vi "M2p_AD_Fifo.vi"() -> ()   [LabVIEW 2015]
uses:
  spcm_library/spcm_gui_common.llb/element_device.ctl
  spcm_library/spcm_gui_common.llb/element_mode_fifo.ctl
  spcm_library/spcm_gui_common.llb/element_device_infos.ctl
  spcm_library/spcm_gui_m2p.llb/element_m2p_ai_channel.ctl
  spcm_library/spcm_gui_m2p.llb/element_m2p_clock.ctl
  spcm_library/spcm_gui_m2p.llb/element_m2p_ai_trigger.ctl
panel:
  out "Display Ch2-Ch3":sgl[][](graph)
  out "Display Ch0-Ch1":sgl[][](graph)
  in  "Trigger Settings":T1={"Trigger Source"=0, "External Trigger"=0, "Level 0 Ext"=1500, "Ext Trig Term"=FALSE, "Channel Trigger"=0, "Level 0 Ch"=0, "Level 1 Ch"=0, "Trigger Delay (Samples)"=0} {"Channel Trigger" items=["None", "Pos. Edge", "Neg. Edge", "Any Edge", "Pos. Rearm", "Neg. Rearm", "Enter Window", "Leave Window", "In Win", "Out Win"]; "External Trigger" items=["None", "Pos. Edge", "Neg. Edge", "Any Edge", "High Level", "Low Level"]; "Trigger Source" items=["Software Trigger", "External Trigger", "Channel 0 Trigger", "Channel 1 Trigger", "Channel 2 Trigger", "Channel 3 Trigger", "Channel 4 Trigger", "Channel 5 Trigger", "Channel 6 Trigger", "Channel 7 Trigger"]; "Trigger Delay (Samples)" max=65535 step=1}
  in  "Clock Settings":T2={"Clock Mode"=0, "Sampling Rate (kHz)"=10000.0, "Clock Output"=FALSE, "Termination"=FALSE, "Ref. Clock (MHz)"=10.0, "Threshold (mV)"=1500} {"Threshold (mV)" min=-5000 max=5000; "Clock Mode" items=["Internal Clock Quartz", "External Clock", "External Reference Clock"]; "Ref. Clock (MHz)" min=0.0 max=125000.0; "Sampling Rate (kHz)" min=1.0 max=5000000.0}
  in  "AI Channel 7":T3={"Enable"=TRUE, "Input Range "=2, "Termination"=0, "Input Type"=0, "Offset"=0} {"Input Type" items=["Single-ended", "Differential"]; "Termination" items=["1 MOhm", "50 Ohm"]; "Input Range" items=["±200 mV", "±500 mV", "±1000 mV", "±2000 mV", "±5000 mV", "±10000 mV"]}
  in  "AI Channel 6":T3={"Enable"=TRUE, "Input Range "=2, "Termination"=0, "Input Type"=0, "Offset"=0} {"Input Type" items=["Single-ended", "Differential"]; "Termination" items=["1 MOhm", "50 Ohm"]; "Input Range" items=["±200 mV", "±500 mV", "±1000 mV", "±2000 mV", "±5000 mV", "±10000 mV"]}
  in  "AI Channel 5":T3={"Enable"=TRUE, "Input Range "=2, "Termination"=0, "Input Type"=0, "Offset"=0} {"Input Type" items=["Single-ended", "Differential"]; "Termination" items=["1 MOhm", "50 Ohm"]; "Input Range" items=["±200 mV", "±500 mV", "±1000 mV", "±2000 mV", "±5000 mV", "±10000 mV"]}
  in  "AI Channel 4":T3={"Enable"=TRUE, "Input Range "=2, "Termination"=0, "Input Type"=0, "Offset"=0} {"Input Type" items=["Single-ended", "Differential"]; "Termination" items=["1 MOhm", "50 Ohm"]; "Input Range" items=["±200 mV", "±500 mV", "±1000 mV", "±2000 mV", "±5000 mV", "±10000 mV"]}
  in  "AI Channel 3":T3={"Enable"=TRUE, "Input Range "=2, "Termination"=0, "Input Type"=0, "Offset"=0} {"Input Type" items=["Single-ended", "Differential"]; "Termination" items=["1 MOhm", "50 Ohm"]; "Input Range" items=["±200 mV", "±500 mV", "±1000 mV", "±2000 mV", "±5000 mV", "±10000 mV"]}
  in  "AI Channel 2":T3={"Enable"=TRUE, "Input Range "=2, "Termination"=0, "Input Type"=0, "Offset"=0} {"Input Type" items=["Single-ended", "Differential"]; "Termination" items=["1 MOhm", "50 Ohm"]; "Input Range" items=["±200 mV", "±500 mV", "±1000 mV", "±2000 mV", "±5000 mV", "±10000 mV"]}
  in  "AI Channel 1":T3={"Enable"=TRUE, "Input Range "=2, "Termination"=0, "Input Type"=0, "Offset"=0} {"Input Type" items=["Single-ended", "Differential"]; "Termination" items=["1 MOhm", "50 Ohm"]; "Input Range" items=["±200 mV", "±500 mV", "±1000 mV", "±2000 mV", "±5000 mV", "±10000 mV"]}
  in  "AI Channel 0":T3={"Enable"=TRUE, "Input Range "=2, "Termination"=0, "Input Type"=0, "Offset"=0} {"Input Type" items=["Single-ended", "Differential"]; "Termination" items=["1 MOhm", "50 Ohm"]; "Input Range" items=["±200 mV", "±500 mV", "±1000 mV", "±2000 mV", "±5000 mV", "±10000 mV"]}
  out "Device Infos":T4={"Device Name"="M2p.5942-x4", "Serial Number"=666.0, "Mem (MB)"=1024.0}
  out "Display Ch6-Ch7":sgl[][](graph)
  out "Display Ch4-Ch5":sgl[][](graph)
  in  "Mode Setup":T5={"Mode"=0, "Loop"=0, "Seg"=1024, "Post"=8192, "Pre"=32, "ABA"=16} {"Mode" items=["Singleshot", "Multiple Recording", "Gated Sampling", "ABA Mode"]; "ABA" min=2 max=65535 step=1; "Post" min=4 step=4; "Loop" min=8 step=4; "Pre" min=4 max=8176 step=4; "Seg" min=8 step=4}
  in  "Device":T6 {"Device" items=["Card", "digitizerNETBOX"]}
  out "Fillsize Fifo":i32(slide)=62 scale=0.0..1000.0
  out "Status":string="Stopped"
  in  "Quit Button":bool
  in  "Force Trigger Button":bool
  in  "Start Button":bool
  in  "Stop Button":bool
  # "M2p AD FIFO Example"
  # "Mode Settings"
  # "Range"
  # "Term"
  # "Type"
  # "Offset"
  # "Ch0"
  # "Ch1"
  # "Clock Settings"
  # "Ch2"
  # "Ch3"
  # "Ch4"
  # "Trigger Settings"
  # "Ch5"
  # "Ch6"
  # "Ch7"
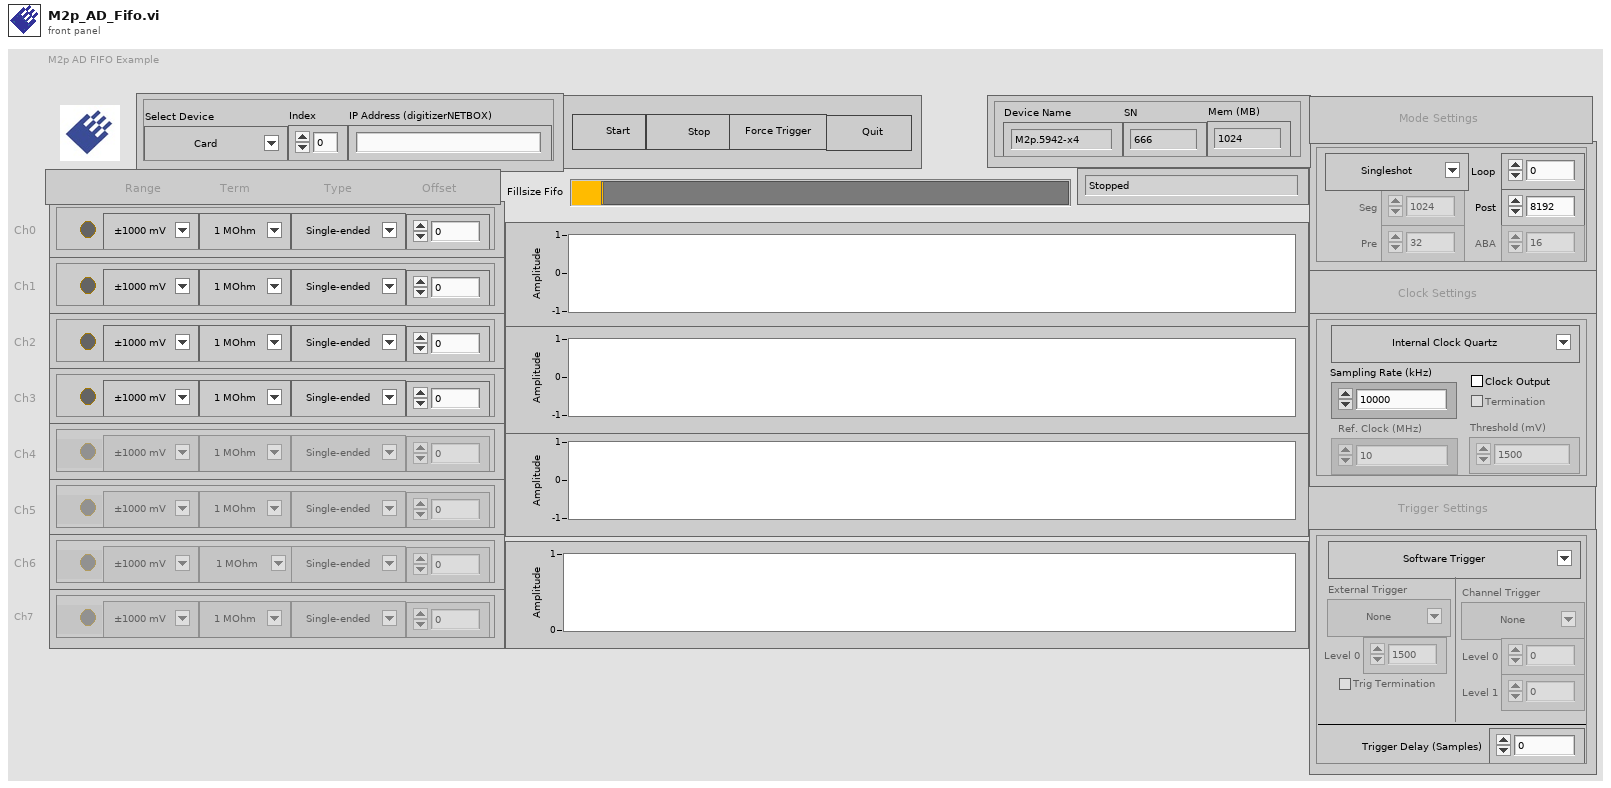
[diagram p1: front panel]
types:
  T1 = typedef "element_m2p_ai_trigger.ctl" = cluster{"Trigger Source":u16, "External Trigger":u16, "Level 0 Ext":i32, "Ext Trig Term":bool, "Channel Trigger":u16, "Level 0 Ch":i32, "Level 1 Ch":i32, "Trigger Delay (Samples)":u32}
  T2 = typedef "element_m2p_clock.ctl" = cluster{"Clock Mode":u16, "Sampling Rate (kHz)":dbl, "Clock Output":bool, "Termination":bool, "Ref. Clock (MHz)":dbl, "Threshold (mV)":i32}
  T3 = typedef "element_m2p_ai_channel.ctl" = cluster{"Enable":bool, "Input Range ":u16, "Termination":u16, "Input Type":u16, "Offset":i32}
  T4 = typedef "element_device_infos.ctl" = cluster{"Device Name":string, "Serial Number":dbl, "Mem (MB)":dbl}
  T5 = typedef "element_mode_fifo.ctl" = cluster{"Mode":u16, "Loop":u32, "Seg":u32, "Post":u32, "Pre":u32, "ABA":u32}
  T6 = typedef "element_device.ctl" = cluster{"Index":dbl, "IP Address":string, "Device":u16}
  T7 = enum16{"Idle", "Init", "Stop", "Write Setup", "Start", "Acquire", "Read Data", "Quit"}
  T8 = cluster{"Card Type":i32, "Inst Mem (high part)":i32, "Inst Mem (low part)":i32, "Serial Number":i32, "Function Type":i32, "Installed Features":i32, "Base Card Version":i32, "Module Version":i32, "Extension Version":i32, "Production Date":i32, "Max Sampling Rate":i32, "Max Channels":i32, "Demo Card":i32}
  T9 = cluster{"Card Name":string, "SN":i32, "Mem (MB)":i32}
  T10 = cluster{"AI Channels":i32, "AI Ranges":i32, "Input Ranges (mV)":i32[], "Programmable Offset":i32, "Termination Available":bool, "SE/Diff switchable":bool, "Offset in per cent/mV":bool, "Offset Calibration":bool, "Gain Calibration":bool, "Offset with open inputs":bool, "AI Range Strings[]":string[], "Bit Resolution":i32, "AC Coupling available":bool, "BW Limit available":bool, "AI Path count":i32}
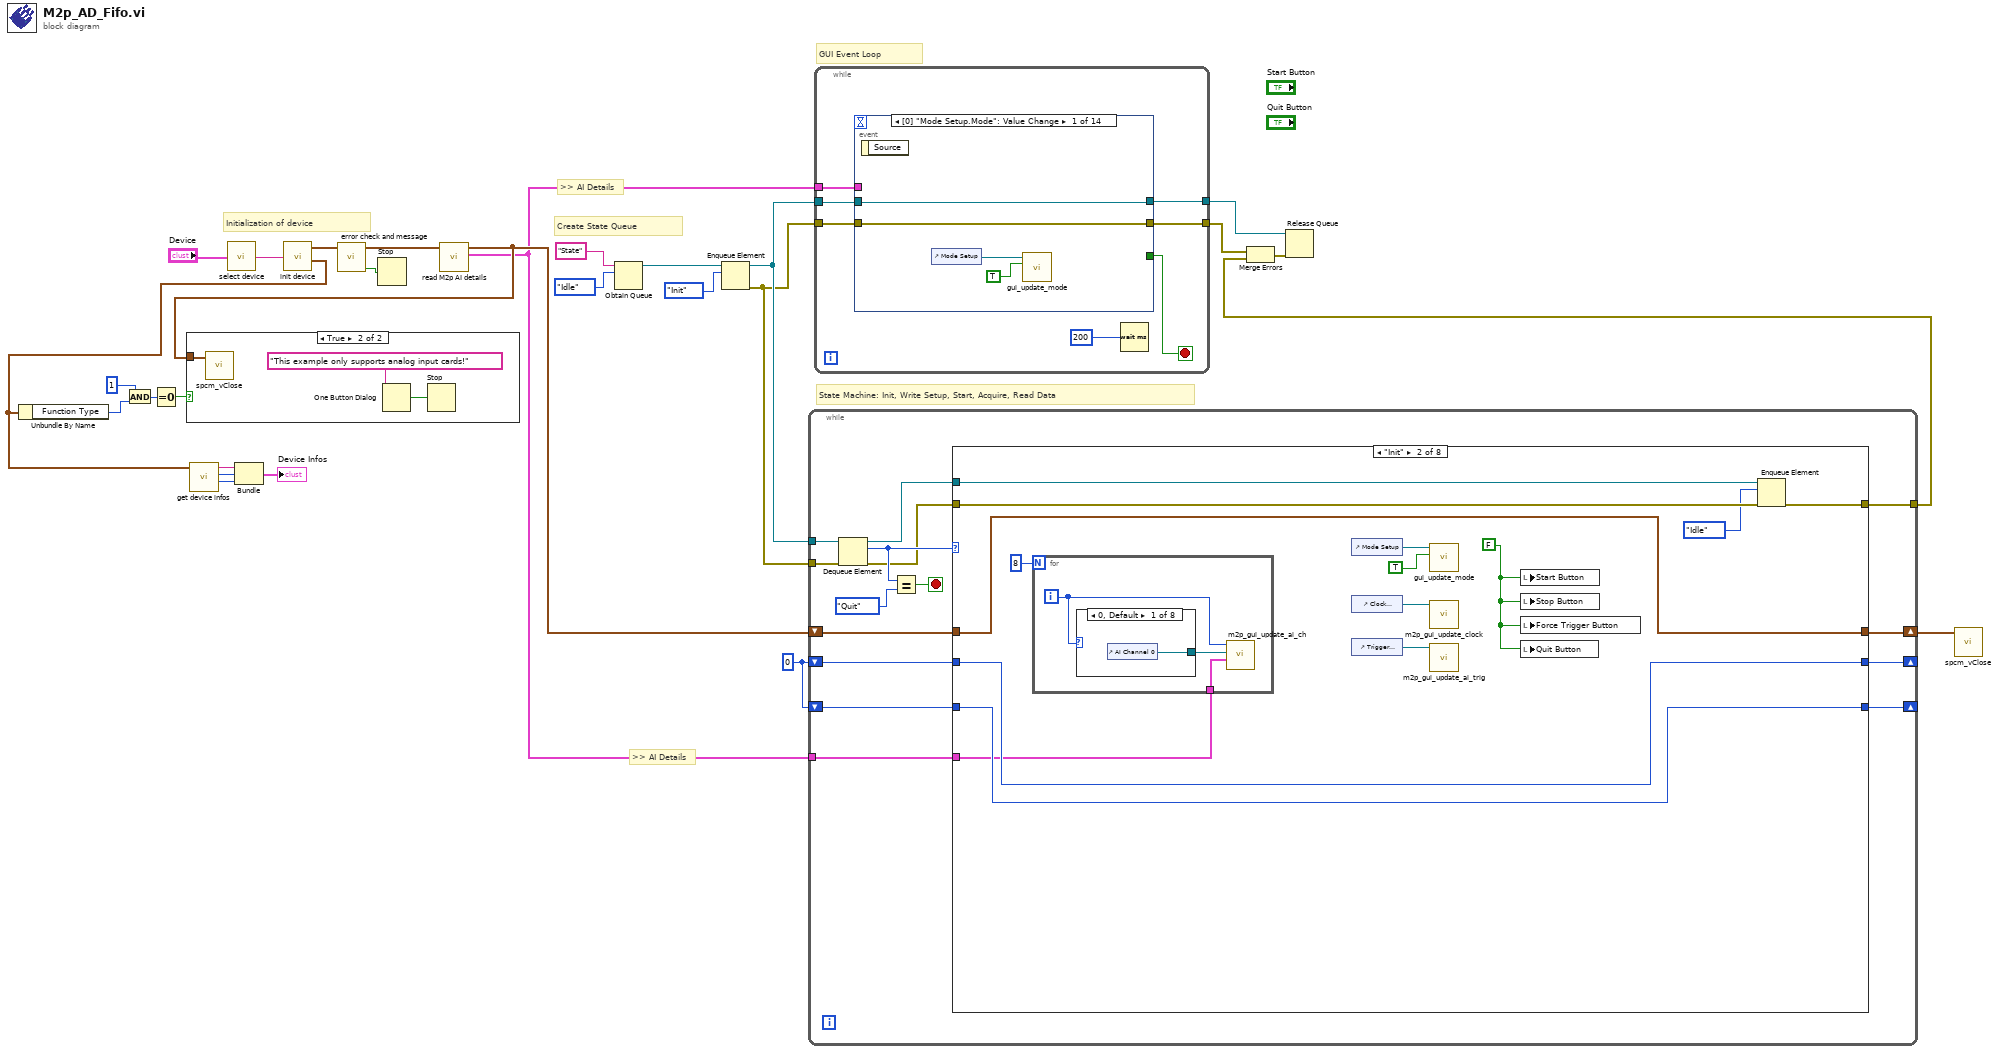
[diagram p0: block diagram]
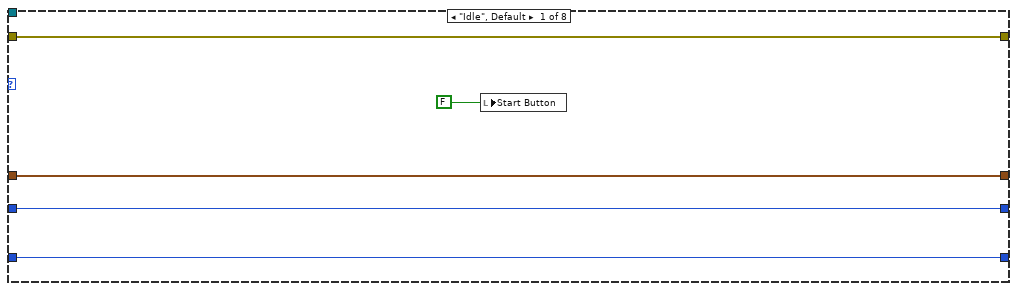
[diagram p3: hidden frame]
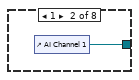
[diagram p4: hidden frame]
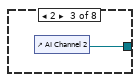
[diagram p5: hidden frame]
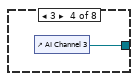
[diagram p6: hidden frame]
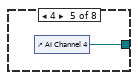
[diagram p7: hidden frame]
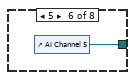
[diagram p8: hidden frame]
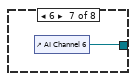
[diagram p9: hidden frame]
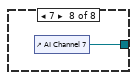
[diagram p10: hidden frame]
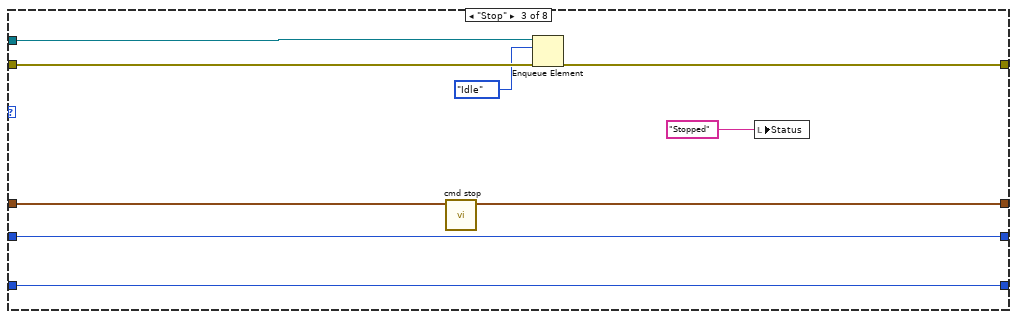
[diagram p11: hidden frame]
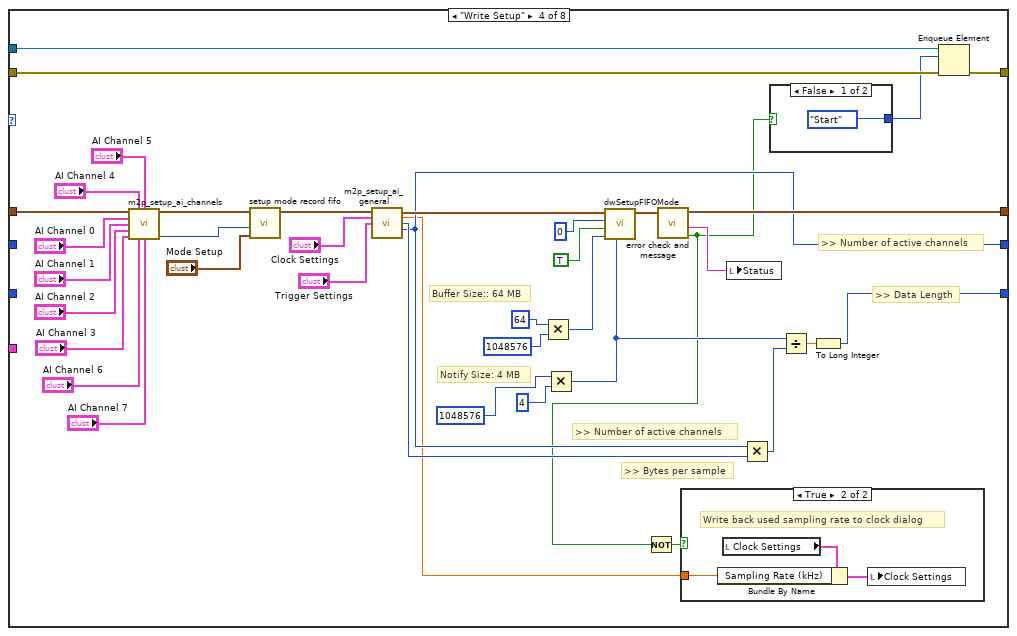
[diagram p12: hidden frame]
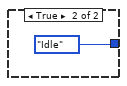
[diagram p14: hidden frame]
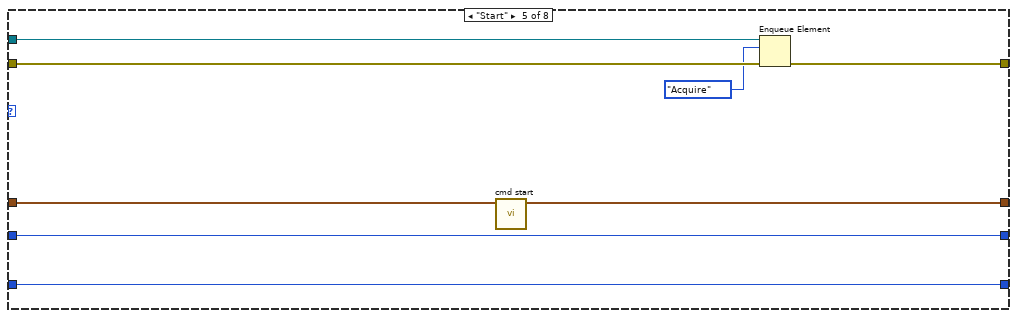
[diagram p15: hidden frame]
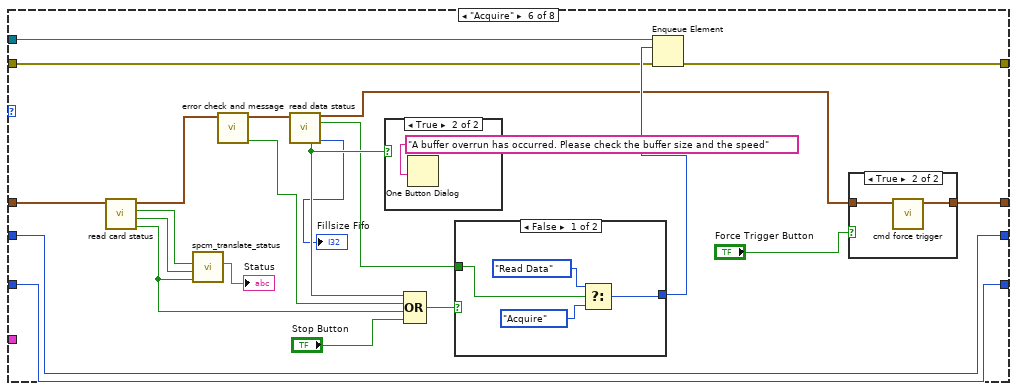
[diagram p16: hidden frame]
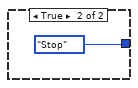
[diagram p18: hidden frame]
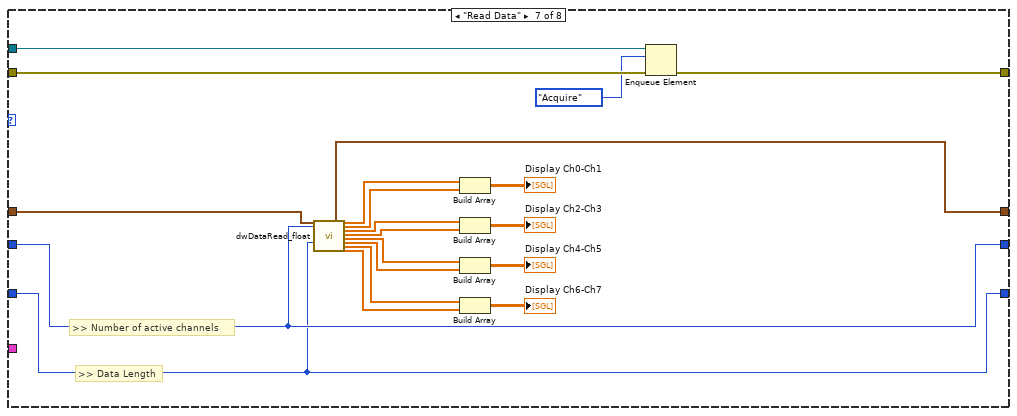
[diagram p20: hidden frame]
diagram:
  w6 = 0
  # ">> AI Details"
  # ">> AI Details"
  # "Initialization of device"
  # "Create State Queue"
  # "State Machine: Init, Write Setup, Start, Acquire, Read Data"
  # "GUI Event Loop"
  n1 = call "select device.vi"("Device"="Device") -> ("device string"=w28:string)  [unwired: 4 in]
  n2 = call "init device.vi"("Device String"=w28) -> ("Card Info Out"=w27:cluster{"Card Handle":u64, "Error Code":u32}, "Card Information"=w14:T8)  [unwired: 4 in]
  n3 = Unbundle By Name(w14) -> ("Function Type"=w18:i32)
  n4 = And(x=1, y=w18) -> (x .and. y?=w17:i32)
  n5 = Equal To 0?(x=w17) -> (x = 0?=w15:bool)
  n6 = call "get device infos.vi"("Card Information"=w14) -> ("Mem (MB)"=w21:i32, "SN"=w20:i32, "Card Name"=w19:string)  [unwired: 8 in]
  n7 = Bundle("Card Name"=w19, "SN"=w20, "Mem (MB)"=w21) -> (→"Device Infos":T9)  [unwired: 1 in]
  n8 = call "error check and message.vi"("Card Info In"=w27) -> ("Error occurred"=w26:bool, "Card Info Out"=w4:cluster{"Card Handle":u64, "Error Code":u32})  [unwired: 4 in, 1 out]
  n9 = Stop(stop? (T)=w26) -> ()
  n10 = call "read M2p AI details.vi"("Card Info In"=w4) -> ("AI Details"=w2:T10, "Card Info Out"=w3:cluster{"Card Handle":u64, "Error Code":u32})  [unwired: 5 in]
  n11 = case shown="True" w15 {
    tunnel: w3 -> [_ w29]
    frame False {
    }
    frame True {
      n12 = call "spcm_vClose.vi"("Card Info In"=w29) -> ()  [unwired: 7 in]
      n13 = One Button Dialog(message="This example only supports analog input cards!") -> (true=w30:bool)  [unwired: 1 in]
      n14 = Stop(stop? (T)=w30) -> ()
    }
  }
  n15 = Obtain Queue(name (unnamed)="State", element data type=T7."Idle") -> (queue out=w23:refnum<queue>)  [unwired: 3 in, 2 out]
  n16 = Enqueue Element(queue=w23, element=T7."Init") -> (queue out=w24:refnum<queue>, error out=w9:errorcluster)  [unwired: 2 in, 1 out]
  n17 = while {
    tunnel: w24 -> [w46]
    shift-right: [w44] -> w22
    shift-left: w3 -> [w45]
    shift-right: [w39] -> _
    shift-left: w6 -> [w40]
    tunnel: [w38] -> w12
    tunnel: w9 -> [w37]
    shift-right: [w34] -> _
    shift-left: w6 -> [w33]
    tunnel: w2 -> [w32]
    stop <- w42 stop-if-true
    n18 = Dequeue Element(queue=w46, error in (no error)=w37) -> (queue out=w41:refnum<queue>, element=w43:T7, error out=w36:errorcluster)  [unwired: 1 in, 1 out]
    n19 = Equal?(x=w43, y=T7."Quit") -> (x = y?=w42:bool)
    n20 = case shown="\"Init\"" w43 {
      tunnel: w45 -> [w51 w58 w82 w99 w136 w149 w187 w190]
      tunnel: [w51 w58 w81 w121 w135 w156 w181 w189] -> w44
      tunnel: w41 -> [_ w65 w85 w124 w133 w154 w188 _]
      tunnel: w40 -> [w50 w59 w80 _ w137 w153 w186 w194]
      tunnel: [w50 w59 w80 w102 w137 w153 w186 w194] -> w39
      tunnel: [w49 w63 w83 w122 w132 w151 w185 w195] -> w38
      tunnel: w36 -> [w49 w62 w84 w123 w134 w150 w184 w195]
      tunnel: [w47 w60 w79 w111 w130 w139 w183 w193] -> w34
      tunnel: w33 -> [w47 w60 w79 _ w130 w139 w183 w193]
      tunnel: w32 -> [_ w55 _ _ _ _ _ _]
      frame "Idle", Default {
        n21 = local write "Start Button"(FALSE) -> ()
      }
      frame "Init" {
        w64 = FALSE
        n22 = for {
          N: 8 -> [_]
          tunnel: w55 -> [w66]
          i -> [w68]
          n23 = case shown="0, Default" w68 {
            tunnel: [w69 w70 w71 w72 w73 w74 w75 w76] -> w67
            frame 0, Default {
              n24 = control-ref of="AI Channel 0"() -> (w69:refnum<vi>)
            }
            frame 1 {
              n25 = control-ref of="AI Channel 1"() -> (w70:refnum<vi>)
            }
            frame 2 {
              n26 = control-ref of="AI Channel 2"() -> (w71:refnum<vi>)
            }
            frame 3 {
              n27 = control-ref of="AI Channel 3"() -> (w72:refnum<vi>)
            }
            frame 4 {
              n28 = control-ref of="AI Channel 4"() -> (w73:refnum<vi>)
            }
            frame 5 {
              n29 = control-ref of="AI Channel 5"() -> (w74:refnum<vi>)
            }
            frame 6 {
              n30 = control-ref of="AI Channel 6"() -> (w75:refnum<vi>)
            }
            frame 7 {
              n31 = control-ref of="AI Channel 7"() -> (w76:refnum<vi>)
            }
          }
          n32 = call "m2p_gui_update_ai_ch.vi"("AI Details"=w66, "Cluster Referenz"=w67, "Channel Index"=w68) -> ()  [unwired: 9 in]
        }
        n33 = control-ref of="Mode Setup"() -> (w57:refnum<vi>)
        n34 = control-ref of="Clock Settings"() -> (w54:refnum<vi>)
        n35 = control-ref of="Trigger Settings"() -> (w53:refnum<vi>)
        n36 = call "gui_update_mode.vi"("Fifo Mode"=TRUE, "Referenz Mode Settings"=w57) -> ()  [unwired: 10 in]
        n37 = call "m2p_gui_update_clock.vi"("Cluster Reference"=w54) -> ()  [unwired: 11 in]
        n38 = call "m2p_gui_update_ai_trig.vi"("Trigger Settings Reference"=w53) -> ()  [unwired: 10 in]
        n39 = local write "Start Button"(w64) -> ()
        n40 = local write "Stop Button"(w64) -> ()
        n41 = local write "Force Trigger Button"(w64) -> ()
        n42 = local write "Quit Button"(w64) -> ()
        n43 = Enqueue Element(queue=w65, element=T7."Idle", error in (no error)=w62) -> (error out=w63:errorcluster)  [unwired: 1 in, 2 out]
      }
      frame "Stop" {
        n44 = call "cmd stop.vi"("Card Info In"=w82) -> ("Card Info Out"=w81:cluster{"Card Handle":u64, "Error Code":u32})  [unwired: 6 in]
        n45 = Enqueue Element(queue=w85, element=T7."Idle", error in (no error)=w84) -> (error out=w83:errorcluster)  [unwired: 1 in, 2 out]
        n46 = local write "Status"("Stopped") -> ()
      }
      frame "Write Setup" {
        # ">> Data Length"
        # ">> Number of active channels"
        # ">> Bytes per sample"
        # ">> Number of active channels"
        # "Buffer Size:: 64 MB"
        # "Notify Size: 4 MB"
        n47 = call "m2p_setup_ai_channels.vi"("Card Info In"=w99, "AI Channel 4"="AI Channel 4", "AI Channel 5"="AI Channel 5", "AI Channel 0"="AI Channel 0", "AI Channel 1"="AI Channel 1", "AI Channel 2"="AI Channel 2", "AI Channel 3"="AI Channel 3", "AI Channel 6"="AI Channel 6", "AI Channel 7"="AI Channel 7") -> ("Card Info Out"=w100:cluster{"Card Handle":u64, "Error Code":u32}, "ChMask"=w90:i32)  [unwired: 5 in]
        n48 = call "setup mode record fifo.vi"("Mode Fifo Setup"="Mode Setup", "Channel Mask Low"=w90, "Card Info In"=w100) -> ("Card Info Out"=w105:cluster{"Card Handle":u64, "Error Code":u32})  [unwired: 2 in, 2 out]
        n49 = call "m2p_setup_ai_general.vi"("Card Info In"=w105, "Clock Settings"="Clock Settings", "Trigger Settings"="Trigger Settings") -> ("Card Info Out"=w104:cluster{"Card Handle":u64, "Error Code":u32}, "Used Sampling Rate (kS)"=w101:dbl, "Bytes Per Sample"=w103:i32, "Channel Count"=w102:i32)  [unwired: 9 in]
        n50 = Multiply(x=u32 64 ("Channel MaskOut"), y=u32 1048576 ("Channel MaskOut")) -> (x*y=w114:u32)
        n51 = Multiply(x=u32 1048576 ("Channel MaskOut"), y=u32 4 ("Channel MaskOut")) -> (x*y=w108:u32)
        n52 = call "dwSetupFIFOMode.vi"("Notify (Bytes)"=w108, "Bufferlength (Bytes)"=w114, "Allocate"=TRUE, "Buffertype (0=data, 1=TS, 2=ABA)"=0, "Card Info In"=w104) -> ("Card Info Out"=w118:cluster{"Card Handle":u64, "Error Code":u32})  [unwired: 4 in]
        n53 = call "error check and message.vi"("Card Info In"=w118) -> ("Error occurred"=w86:bool, "Error Message"=w119:string, "Card Info Out"=w121:cluster{"Card Handle":u64, "Error Code":u32})  [unwired: 4 in]
        n54 = Not(x=w86) -> (.not. x?=w87:bool)
        n55 = case shown="True" w87 {
          tunnel: w101 -> [_ w127]
          frame False {
          }
          frame True {
            # "Write back used sampling rate to clock dialog"
            n56 = local read "Clock Settings"() -> (w126:T2)
            n57 = Bundle By Name(cluster=w126, "Sampling Rate (kHz)"=w127) -> (w125:T2)
            n58 = local write "Clock Settings"(w125) -> ()
          }
        }
        n59 = local write "Status"(w119) -> ()
        n60 = Multiply(x=w102, y=w103) -> (x*y=w113:i32)
        n61 = case shown="False" w86 {
          tunnel: [T7."Start" T7."Idle"] -> w120
          frame False {
          }
          frame True {
          }
        }
        n62 = Divide(x=w108, y=w113) -> (x/y=w112:dbl)
        n63 = To Long Integer(number=w112) -> (32bit integer=w111:i32)
        n64 = Enqueue Element(queue=w124, element=w120, error in (no error)=w123) -> (error out=w122:errorcluster)  [unwired: 1 in, 2 out]
      }
      frame "Start" {
        n65 = call "cmd start.vi"("Card Info In"=w136) -> ("Card Info Out"=w135:cluster{"Card Handle":u64, "Error Code":u32})  [unwired: 6 in]
        n66 = Enqueue Element(queue=w133, element=T7."Acquire", error in (no error)=w134) -> (error out=w132:errorcluster)  [unwired: 1 in, 2 out]
      }
      frame "Acquire" {
        n67 = call "read card status.vi"("Card Info In"=w149) -> ("Card ready"=w141:bool, "Trigger detected"=w158:bool, "Pretrigger full"=w159:bool, "Card Info Out"=w148:cluster{"Card Handle":u64, "Error Code":u32})  [unwired: 3 in]
        n68 = call "spcm_translate_status.vi"("Ready"=w141, "Trigger"=w158, "Pretrigger"=w159) -> ("Text"=→"Status":string)  [unwired: 4 in]
        n69 = call "error check and message.vi"("Card Info In"=w148) -> ("Error occurred"=w143:bool, "Card Info Out"=w147:cluster{"Card Handle":u64, "Error Code":u32})  [unwired: 4 in, 1 out]
        n70 = call "read data status.vi"("Card Info In"=w147) -> ("Card Info Out"=w146:cluster{"Card Handle":u64, "Error Code":u32}, "Next block ready"=w140:bool, "Overrun"=w144:bool, "Fillsize o/oo"=→"Fillsize Fifo":i32)  [unwired: 10 in, 1 out]
        n71 = case shown="True" w144 {
          frame False {
          }
          frame True {
            n72 = One Button Dialog(message="A buffer overrun has occurred. Please check the buffer size and the speed") -> ()  [unwired: 1 in, 1 out]
          }
        }
        n73 = Compound Arithmetic op=OR(w144, w143, w141, "Stop Button") -> (w145:bool)
        n74 = case shown="False" w145 {
          tunnel: [w161 T7."Stop"] -> w157
          tunnel: w140 -> [w164 _]
          frame False {
            n75 = Select(t=T7."Read Data", s=w164, f=T7."Acquire") -> (s? t:f=w161:T7)
          }
          frame True {
          }
        }
        n76 = Enqueue Element(queue=w154, element=w157, error in (no error)=w150) -> (error out=w151:errorcluster)  [unwired: 1 in, 2 out]
        n77 = case shown="True" "Force Trigger Button" {
          tunnel: w146 -> [w166 w168]
          tunnel: [w166 w167] -> w156
          frame False {
          }
          frame True {
            n78 = call "cmd force trigger.vi"("Card Info In"=w168) -> ("Card Info Out"=w167:cluster{"Card Handle":u64, "Error Code":u32})  [unwired: 6 in]
          }
        }
      }
      frame "Read Data" {
        # ">> Data Length"
        # ">> Number of active channels"
        n79 = call "dwDataRead_float.vi"("Card Info In"=w187, "Channel Count"=w186, "Length (Samples per Channel)"=w183) -> ("Card Info Out"=w181:cluster{"Card Handle":u64, "Error Code":u32}, "Ch 0"=w178:sgl[], "Ch 1"=w177:sgl[], "Ch 2"=w176:sgl[], "Ch 3"=w175:sgl[], "Ch 4"=w174:sgl[], "Ch 5"=w173:sgl[], "Ch 6"=w172:sgl[], "Ch 7"=w171:sgl[])  [unwired: 8 in, 8 out]
        n80 = Build Array(w178, w177) -> (→"Display Ch0-Ch1":sgl[][])
        n81 = Build Array(w176, w175) -> (→"Display Ch2-Ch3":sgl[][])
        n82 = Build Array(w174, w173) -> (→"Display Ch4-Ch5":sgl[][])
        n83 = Build Array(w172, w171) -> (→"Display Ch6-Ch7":sgl[][])
        n84 = Enqueue Element(queue=w188, element=T7."Acquire", error in (no error)=w184) -> (error out=w185:errorcluster)  [unwired: 1 in, 2 out]
      }
      frame "Quit" {
        n85 = call "dwSetupFIFOMode.vi"("Allocate"=FALSE, "Buffertype (0=data, 1=TS, 2=ABA)"=0, "Card Info In"=w190) -> ("Card Info Out"=w189:cluster{"Card Handle":u64, "Error Code":u32})  [unwired: 6 in]
      }
    }
  }
  n86 = while {
    tunnel: w24 -> [w200]
    tunnel: [w201] -> w10
    tunnel: [w197] -> w13
    tunnel: w9 -> [w198]
    tunnel: w2 -> [w196]
    stop <- w199 stop-if-true
    n87 = event shown="[0] \"Mode Setup.Mode\": Value Change" {
      selector: _ -> [_ _ _ _ _ _ _ _ _ _ _ _ _ _]
      dyn-events: _ -> [_ _ _ _ _ _ _ _ _ _ _ _ _ _]
      timeout: _ -> [_ _ _ _ _ _ _ _ _ _ _ _ _ _]
      tunnel: [_ _ _ _ _ _ _ _ _ _ _ _ _ TRUE] -> w199
      tunnel: [w206 w209 w212 w217 w222 w227 w232 _ _ _ _ w249 w255 w260] -> w201
      tunnel: w200 -> [w206 w209 w212 w217 w222 w227 w232 _ _ _ _ w248 w254 w261]
      tunnel: [w205 w208 w211 w216 w221 w226 w231 _ _ _ _ w246 w251 w258] -> w197
      tunnel: w198 -> [w205 w208 w211 w216 w221 w226 w231 _ _ _ _ w247 w252 w257]
      tunnel: w196 -> [_ _ _ w213 w218 w223 w228 w233 w236 w239 w242 _ _ _]
      event Value Change {
        n88 = event-data ("Ereignisdatenknoten")() -> ()  [unwired: 1 in, 1 out]
        n89 = control-ref of="Mode Setup"() -> (w204:refnum<vi>)
        n90 = call "gui_update_mode.vi"("Fifo Mode"=TRUE, "Referenz Mode Settings"=w204) -> ()  [unwired: 10 in]
      }
      event Value Change {
        n91 = event-data() -> ()  [unwired: 1 in, 1 out]
        n92 = control-ref of="Clock Settings"() -> (w207:refnum<vi>)
        n93 = call "m2p_gui_update_clock.vi"("Cluster Reference"=w207) -> ()  [unwired: 11 in]
      }
      event Value Change {
        n94 = event-data() -> ()  [unwired: 1 in, 1 out]
        n95 = control-ref of="Trigger Settings"() -> (w210:refnum<vi>)
        n96 = call "m2p_gui_update_ai_trig.vi"("Trigger Settings Reference"=w210) -> ()  [unwired: 10 in]
      }
      event Value Change {
        n97 = event-data() -> ()  [unwired: 1 in, 1 out]
        n98 = control-ref of="AI Channel 0"() -> (w214:refnum<vi>)
        n99 = call "m2p_gui_update_ai_ch.vi"("AI Details"=w213, "Cluster Referenz"=w214, "Channel Index"=0) -> ()  [unwired: 9 in]
      }
      event Value Change {
        n100 = event-data() -> ()  [unwired: 1 in, 1 out]
        n101 = control-ref of="AI Channel 1"() -> (w219:refnum<vi>)
        n102 = call "m2p_gui_update_ai_ch.vi"("AI Details"=w218, "Cluster Referenz"=w219, "Channel Index"=1) -> ()  [unwired: 9 in]
      }
      event Value Change {
        n103 = event-data() -> ()  [unwired: 1 in, 1 out]
        n104 = control-ref of="AI Channel 2"() -> (w224:refnum<vi>)
        n105 = call "m2p_gui_update_ai_ch.vi"("AI Details"=w223, "Cluster Referenz"=w224, "Channel Index"=2) -> ()  [unwired: 9 in]
      }
      event Value Change {
        n106 = event-data() -> ()  [unwired: 1 in, 1 out]
        n107 = control-ref of="AI Channel 3"() -> (w229:refnum<vi>)
        n108 = call "m2p_gui_update_ai_ch.vi"("AI Details"=w228, "Cluster Referenz"=w229, "Channel Index"=3) -> ()  [unwired: 9 in]
      }
      event Value Change {
        n109 = event-data() -> ()  [unwired: 1 in, 1 out]
        n110 = control-ref of="AI Channel 4"() -> (w234:refnum<vi>)
        n111 = call "m2p_gui_update_ai_ch.vi"("AI Details"=w233, "Cluster Referenz"=w234, "Channel Index"=4) -> ()  [unwired: 9 in]
      }
      event Value Change {
        n112 = event-data() -> ()  [unwired: 1 in, 1 out]
        n113 = control-ref of="AI Channel 5"() -> (w237:refnum<vi>)
        n114 = call "m2p_gui_update_ai_ch.vi"("AI Details"=w236, "Cluster Referenz"=w237, "Channel Index"=5) -> ()  [unwired: 9 in]
      }
      event Value Change {
        n115 = event-data() -> ()  [unwired: 1 in, 1 out]
        n116 = control-ref of="AI Channel 6"() -> (w240:refnum<vi>)
        n117 = call "m2p_gui_update_ai_ch.vi"("AI Details"=w239, "Cluster Referenz"=w240, "Channel Index"=6) -> ()  [unwired: 9 in]
      }
      event Value Change {
        n118 = event-data() -> ()  [unwired: 1 in, 1 out]
        n119 = control-ref of="AI Channel 7"() -> (w243:refnum<vi>)
        n120 = call "m2p_gui_update_ai_ch.vi"("AI Details"=w242, "Cluster Referenz"=w243, "Channel Index"=7) -> ()  [unwired: 9 in]
      }
      event "Start Button": Value Change {
        n121 = event-data() -> ()  [unwired: 1 in, 1 out]
        n122 = Enqueue Element(queue=w248, element=T7."Write Setup", error in (no error)=w247) -> (queue out=w249:refnum<queue>, error out=w246:errorcluster)  [unwired: 1 in, 1 out]
      }
      event "Stop Button": Value Change {
        n123 = event-data() -> ()  [unwired: 1 in, 1 out]
        n124 = local write "Start Button"(FALSE) -> ()
        n125 = Enqueue Element(queue=w254, element=T7."Stop", error in (no error)=w252) -> (queue out=w255:refnum<queue>, error out=w251:errorcluster)  [unwired: 1 in, 1 out]
      }
      event "Quit Button": Value Change {
        n126 = event-data() -> ()  [unwired: 1 in, 1 out]
        n127 = Enqueue Element(queue=w261, element=T7."Quit", error in (no error)=w257) -> (queue out=w260:refnum<queue>, error out=w258:errorcluster)  [unwired: 1 in, 1 out]
      }
    }
    n128 = Wait (ms)(milliseconds to wait=200) -> ()  [unwired: 1 out]
  }
  n129 = Merge Errors(w13, w12) -> (w11:errorcluster)
  n130 = Release Queue(queue=w10, error in (no error)=w11) -> ()  [unwired: 1 in, 3 out]
  n131 = call "spcm_vClose.vi"("Card Info In"=w22) -> ()  [unwired: 7 in]
